vi "Finish.vi"(8 "error in (no error)":errorcluster, 11 "One Driver in":refnum<class "One Driver.lvclass">) -> (0 "error out":errorcluster, 3 "One Driver out":refnum<class "One Driver.lvclass">)   [LabVIEW 2019, in "Joysticks.lvlib" / "One Driver.lvclass"]
doc: "Use this method to close the references to the joysticks."
uses:
  One Driver.lvclass
  One Driver.lvclass/One Driver.ctl
  <vilib>/Rock Robotics/WPI/Utilities/WPI_GetSetVariantRefNum.vi
  Joysticks.lvclass
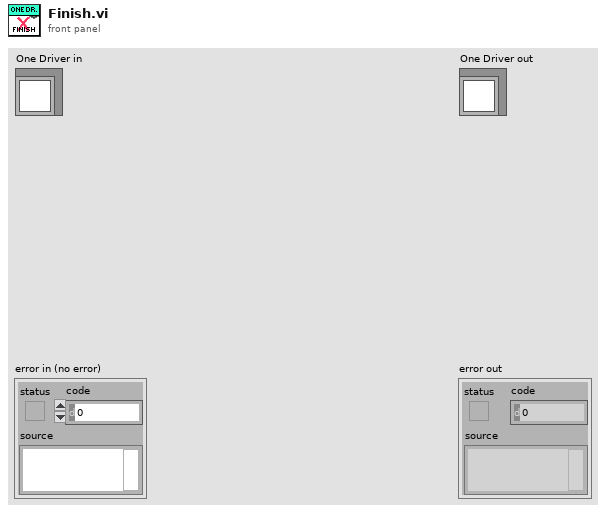
[diagram p1: front panel]
types:
  T1 = typedef "WPI_JoystickDevRef.ctl" = cluster{"Device":T2}
  T2 = typedef "WPI_JoystickDeviceEnum.ctl" = enum16{"USB 0", "USB 1", "USB 2", "USB 3", "USB 4", "USB 5"}
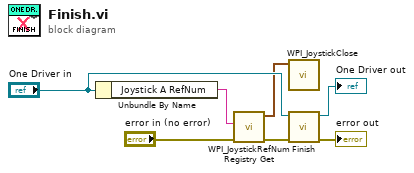
[diagram p0: block diagram]
diagram:
  n1 = Unbundle By Name("One Driver in") -> ("Joystick A RefNum"=w3:string)
  n2 = call <vilib>:"WPI_JoystickRefNum Registry Get.vi"("error in (no error)"="error in (no error)", "refnum name"=w3) -> ("error out"=w1:errorcluster, "JoystickDevRef"=w2:T1)  [unwired: 8 in]
  n3 = call <vilib>:"WPI_JoystickClose.vi"("JoystickDevRef"=w2) -> ()  [unwired: 11 in]
  n4 = call-parent "Finish.vi"("error in (no error)"=w1, "Joysticks in"="One Driver in") -> ("error out"=→"error out":errorcluster, "Joysticks out"=→"One Driver out":refnum<class "One Driver.lvclass">)  [unwired: 8 in]
